vi "UFF_ReadFile.vi"(11 "file (use dialog)":path) -> (2 "packets":string[](array[string]), 3 "text":string)   [LabVIEW 2022 SP3]
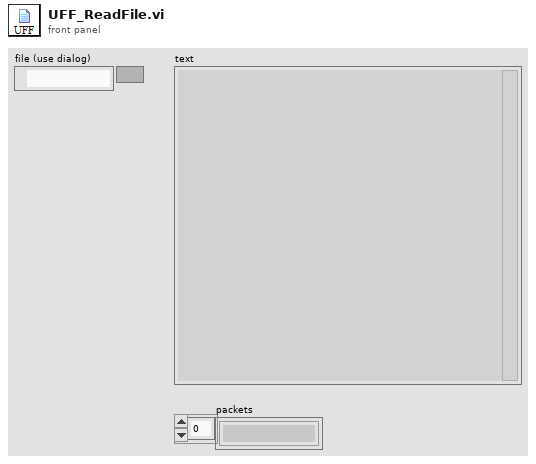
[diagram p1: front panel]
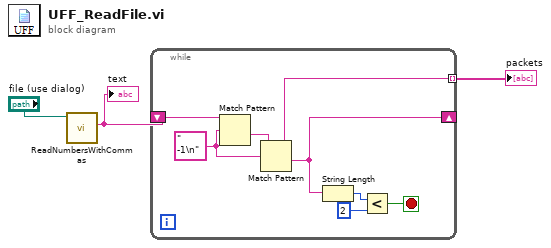
[diagram p0: block diagram]
diagram:
  n1 = call "ReadNumbersWithCommas.vi"("file (use dialog)"="file (use dialog)") -> ("text"=w2:string)  [unwired: 7 in, 3 out]
  "text" <- w2
  n2 = while {
    shift-right: [w7] -> _
    shift-left: w2 -> [w11]
    tunnel: [w8] -> w3 mode=indexing
    stop <- w4 stop-if-true
    w9 = "    -1\n" ("regular expression")
    n3 = Match Pattern(string=w11, regular expression=w9) -> (after substring=w10:string)  [unwired: 1 in, 3 out]
    n4 = Match Pattern(string=w10, regular expression=w9) -> (before substring=w8:string, after substring=w7:string)  [unwired: 1 in, 2 out]
    n5 = String Length(string=w7) -> (length=w6:i32)
    n6 = Less?(x=w6, y=2) -> (x < y?=w4:bool)
  }
  "packets" <- w3
